vi "insertion sorting.vi"(2 "values between 1~10000":dbl[](array[numeric]), 4 "N numbers":i32) -> ()   [LabVIEW 2014]
panel:
  out "Insertion Sort":dbl[](graph)
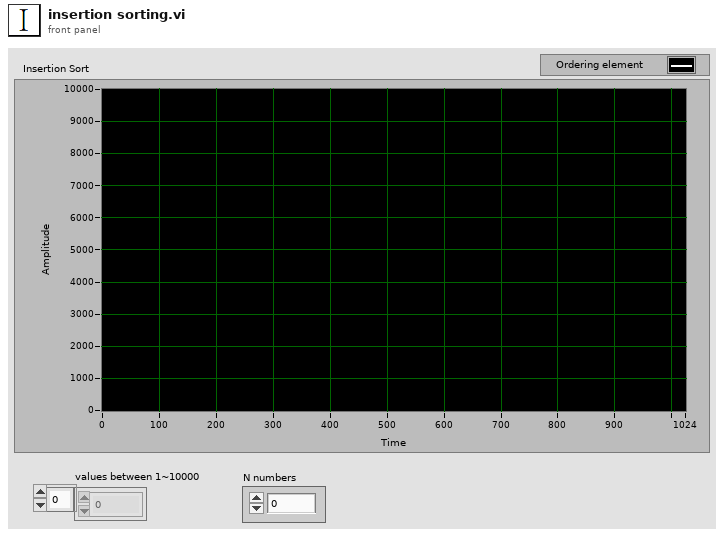
[diagram p1: front panel]
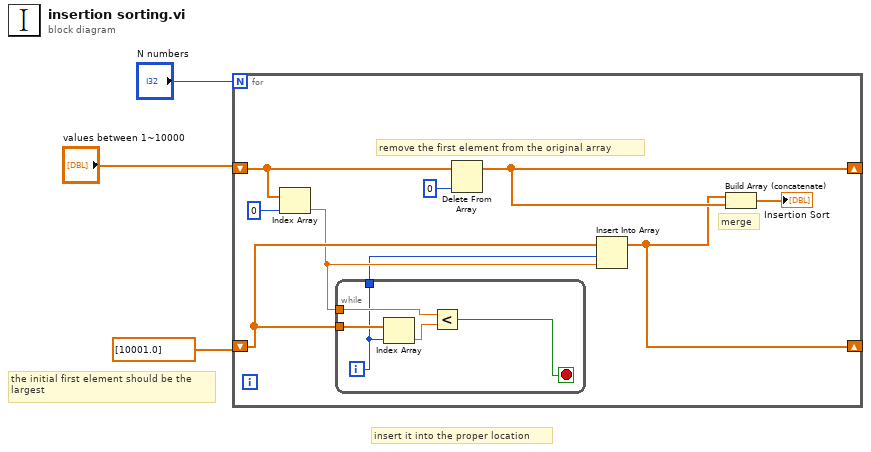
[diagram p0: block diagram]
diagram:
  # "the initial first element should be the\nlargest"
  # "insert it into the proper location"
  n1 = for {
    N: "N numbers" -> [_]
    shift-right: [w7] -> _
    shift-left: "values between 1~10000" -> [w11]
    shift-right: [w4] -> _
    shift-left: dbl[] [10001.0] -> [w9]
    # "merge"
    # "remove the first element from the original array"
    n2 = Index Array(array=w11, index=0) -> (element=w8:dbl)
    n3 = while {
      tunnel: w9 -> [w17]
      tunnel: w8 -> [w15]
      tunnel: [w13] -> w5
      i -> [w13]
      stop <- w14 stop-if-true
      n4 = Index Array(array=w17, index=w13) -> (element=w16:dbl)
      n5 = Less?(x=w15, y=w16) -> (x < y?=w14:bool)
    }
    n6 = Delete From Array(array=w11, index=0) -> (array with subset deleted=w7:dbl[])  [unwired: 1 in, 1 out]
    n7 = Insert Into Array(array=w9, index=w5, new element=w8) -> (w4:dbl[])
    n8 = Build Array (concatenate)(w4, w7) -> (→"Insertion Sort":dbl[])
  }
